vi "Format Execution System String.vi"(11 "Preferred Exec System":T1(ring)) -> (3 "Preferred Exec System String":string)   [LabVIEW 2020, in "VI Properties Editor.lvlib"]
doc: "Formats the preferred execution system property into a string to be displayed."
uses:
  VI Properties Editor.lvlib
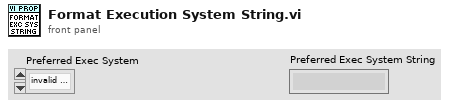
[diagram p1: front panel]
types:
  T1 = enum32{"invalid execution system", "user interface", "standard", "instrument i/o", "data acquisition", "other 1", "other 2", "same as caller"}
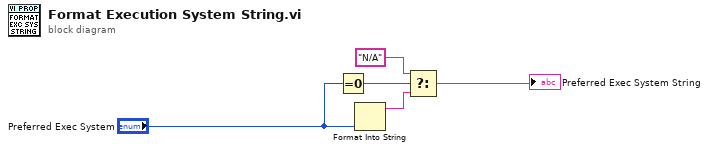
[diagram p0: block diagram]
diagram:
  n1 = Equal To 0?(x="Preferred Exec System") -> (x = 0?=w4:bool)
  n2 = Format Into String("Preferred Exec System") -> (resulting string=w5:string)  [unwired: 3 in, 1 out]
  n3 = Select(t="N/A", s=w4, f=w5) -> (s? t:f=→"Preferred Exec System String":string)
